vi "tester.vi"   [LabVIEW 2020, in "Method Generation.lvlib" / "New Getter Dialog.lvclass"]
uses:
  New Getter Dialog.lvclass
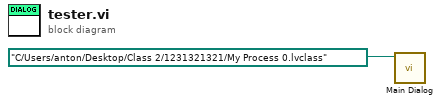
[diagram p0: block diagram]
diagram:
  n1 = call "Main Dialog.vi"("Process Path"=path "C:/Users/anton/Desktop/Class 2/1231321321/My Process 0.lvclass" ("class path")) -> ()  [unwired: 11 in]
